vi "format ANSI SQL wildcards.vi"(3 "String":string) -> (0 "ANSI SQL Wildcard String":string)   [LabVIEW 2011]
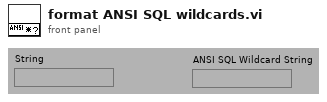
[diagram p1: front panel]
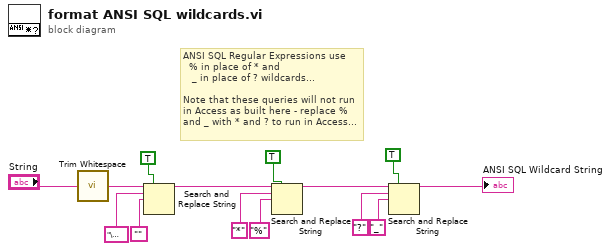
[diagram p0: block diagram]
diagram:
  # "ANSI SQL Regular Expressions use\n  % in place of * and\n   _ in place of ? wildcards...\n\nNote that these queries will not run\nin Access as built here - replace %\nand _ with * and ? to run in Access..."
  n1 = call <vilib>:"Trim Whitespace.vi"("string"="String") -> ("trimmed string"=w7:string)  [unwired: 1 in]
  n2 = Search and Replace String(replace all?=TRUE ("replace all? (F)"), input string=w7, search string="\u0000", replace string="") -> (result string=w4:string)  [unwired: 1 in, 6 out]
  n3 = Search and Replace String(replace all?=TRUE, input string=w4, search string="*", replace string="%" ("string")) -> (result string=w13:string)  [unwired: 1 in, 6 out]
  n4 = Search and Replace String(replace all?=TRUE, input string=w13, search string="?", replace string="_" ("search string")) -> (result string=→"ANSI SQL Wildcard String":string)  [unwired: 1 in, 6 out]
